vi "Get size.vi"(8 "error in (no error)":errorcluster, 11 "system object in":refnum<class "system object.lvclass">) -> (0 "error out":errorcluster, 2 "size":i32, 3 "system object out":refnum<class "system object.lvclass">)   [LabVIEW 2020, in "system object.lvclass"]
uses:
  system object.lvclass
  system object.lvclass/system object.ctl
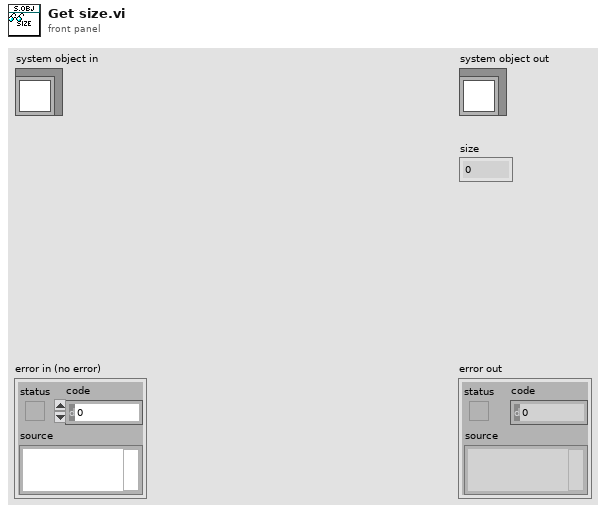
[diagram p1: front panel]
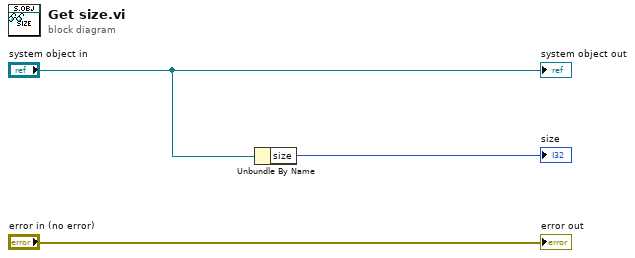
[diagram p0: block diagram]
diagram:
  n1 = Unbundle By Name("system object in") -> ("size"=→"size":i32)
  "error out" <- "error in (no error)"
  "system object out" <- "system object in"
